vi "RT Simulator.vi"() -> ()   [LabVIEW 2015]
uses:
  Type/RT Loop Events.ctl
  Type/TCP Packet Info.ctl
  Type/_RT Command.ctl
panel:
  out "ms Between Commands":u32
  in  "Stop Button":bool
  out "Read Error":errorcluster
  out "Status":string="PC Communication Established"
  out "Time (s)":dbl
  out "Fault":bool
  out "Ready":bool
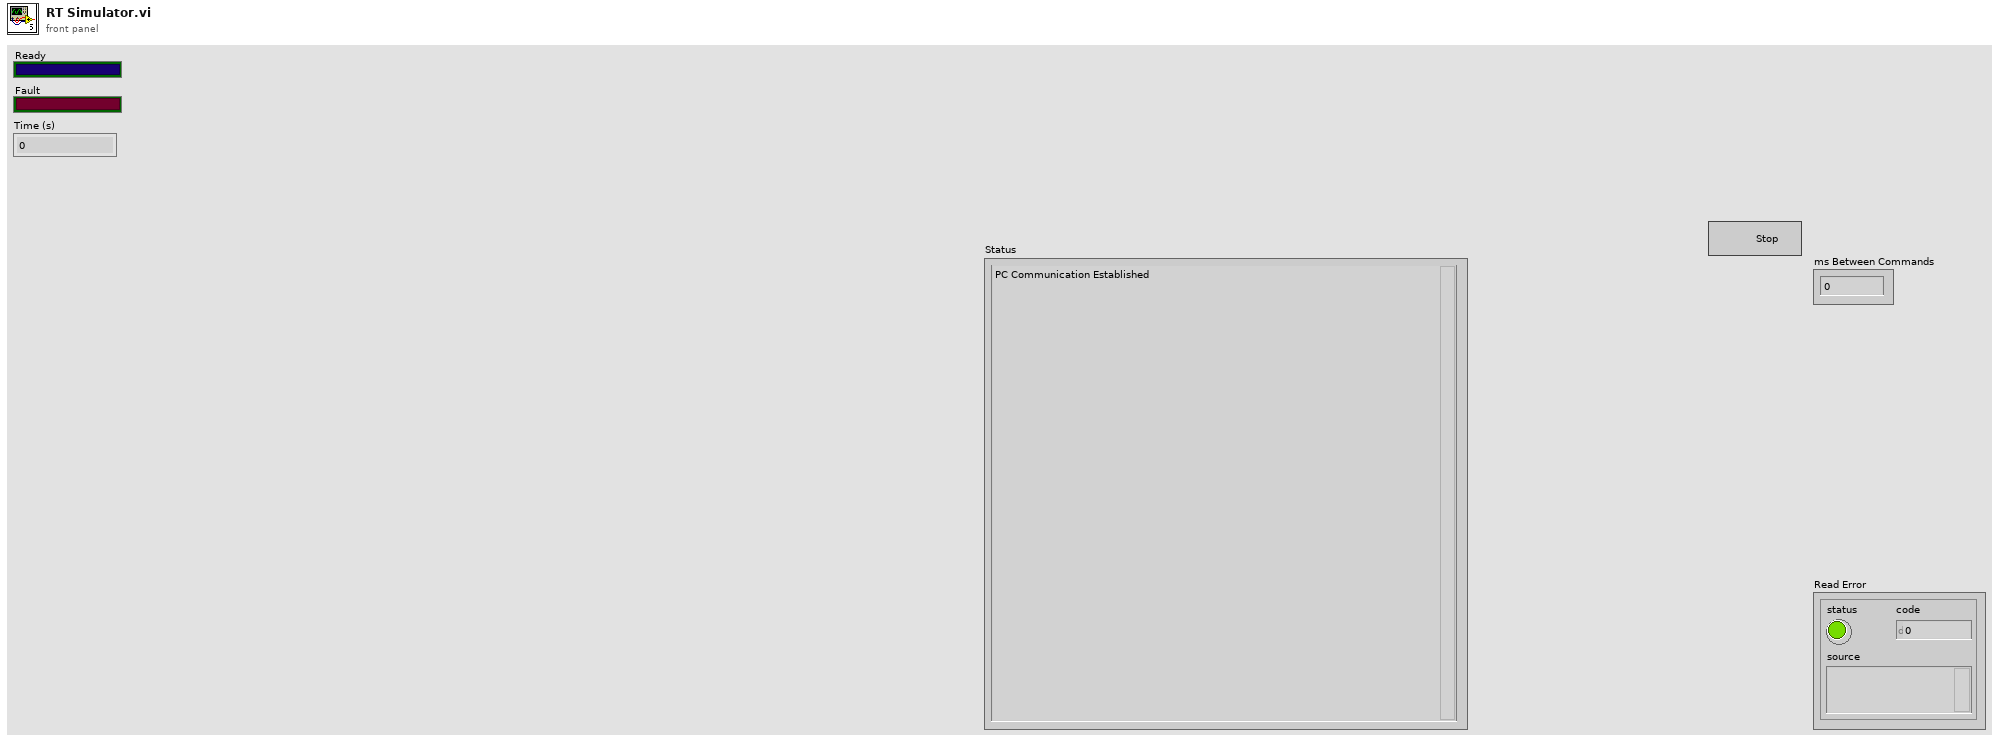
[diagram p1: front panel]
types:
  T1 = typedef "TCP Packet Info.ctl" = cluster{"Packet Signature":string, "Sequence Number":i32, "Command":T2, "Data Message Size":u32, "Data Message Size":string, "Data Message":string, "Error Message Size":u32, "Error Message Size":string, "Error Message":string, "Checksum":u32, "Error Message":errorcluster, "Command ID":string}
  T2 = typedef "_RT Command.ctl" = enum16{"xml Start Run", "xml Start Actual Run", "xml Stop Run", "xml Runtime Update", "xml Get Status", "xml Get Table", "xml Set Table", "xml Get Configuration", "xml System Status", "xml Set LC Input Logic", "xml Get Data", "xml Get Info", "Start", "StartActualRun", "Stop", "Runtime Update", "Get Data", "Get Info", "Get Status", "Get Param", "Get Config", "Get Table", "Read ADC", "Set Oscillator", "Update Config", "Update Table", "Set All Pol", "Set Pol and DC", "Set Max Mass", "Toggle RP", "Toggle EL", "Set PIC", "Initialize Turbo", "Send Turbo Comm", "Close Turbo", "P1", "P2", "P3", "Send Serial", "Set LC Out", "Get LC In", "Read VAC", "Test Table", "Toggle Power", "Get Startup", "Set Startup", "Get ADC Table", "Set ADC Table", "Get Brief Status", "Get Detail Status", "Auxiliary Update", "Set CC Logics", "Set CC Input Logics", "Ignore Error", "invalid"}
  T3 = typedef "RT Loop Events.ctl" = enum16{"Initialize", "Wait for Connection", "Wait for Command", "Send Reply"}
  T4 = cluster{"Rt Loop Events":T3, "Connection ID":refnum<k5>, "error":errorcluster, "Packet Info":T1, "Event":string}
  T5 = enum16{"big-endian, network order", "native, host order", "little-endian"}
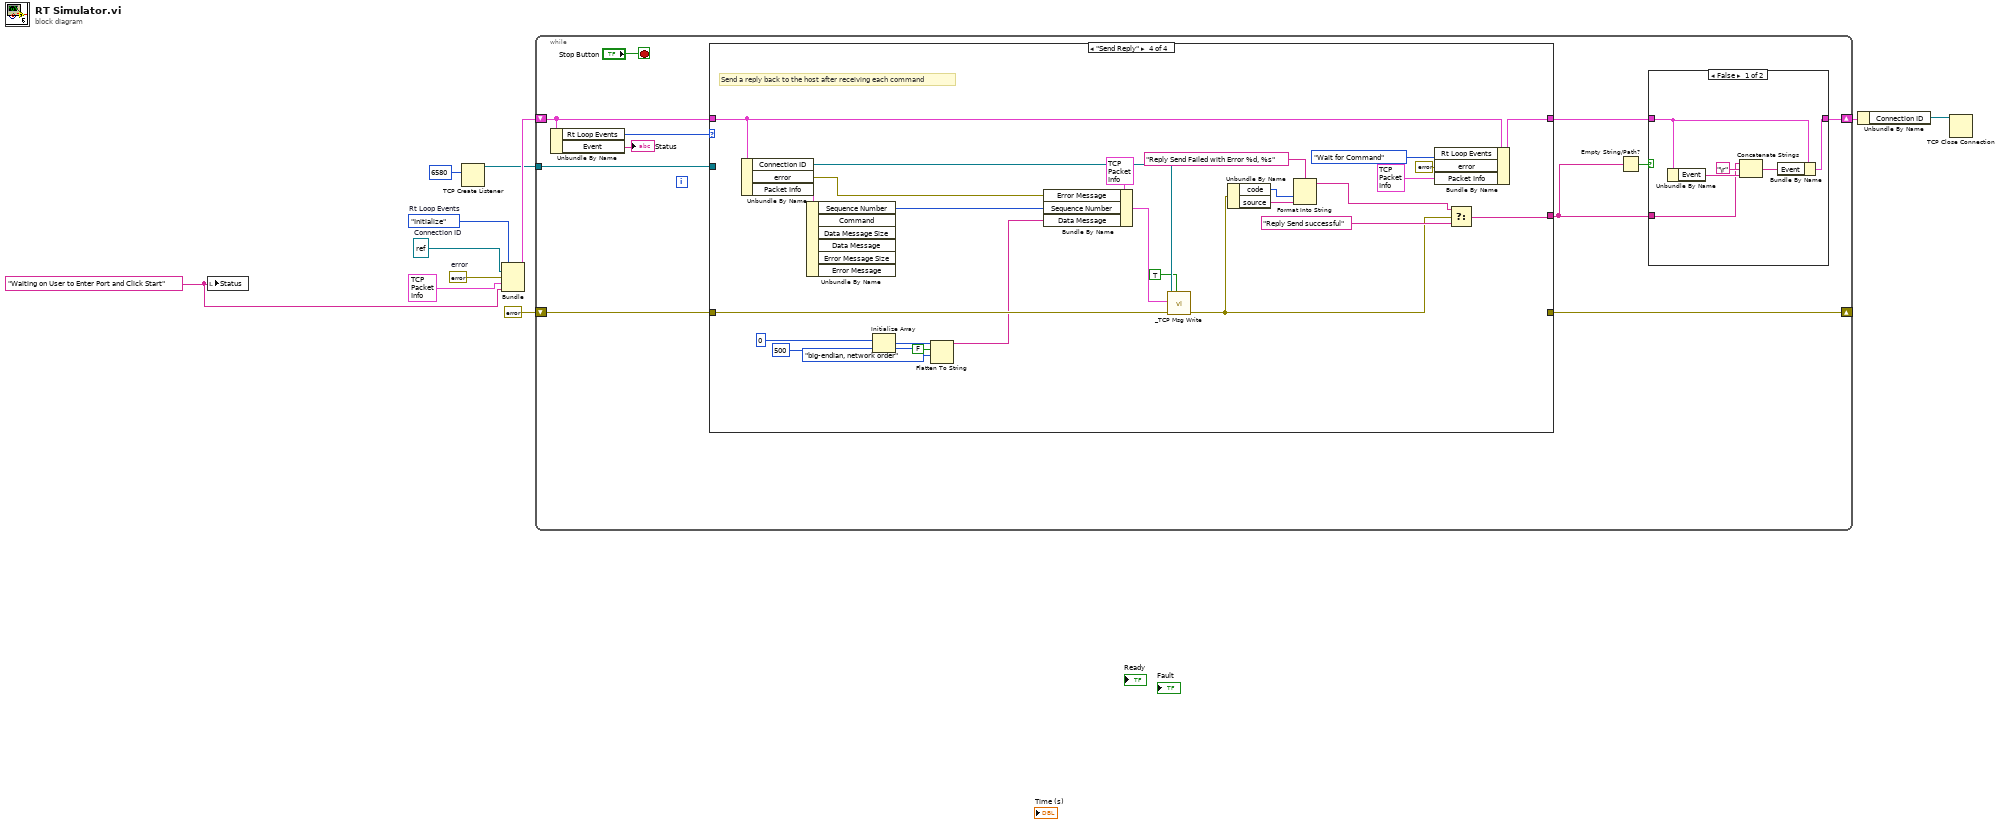
[diagram p0: block diagram]
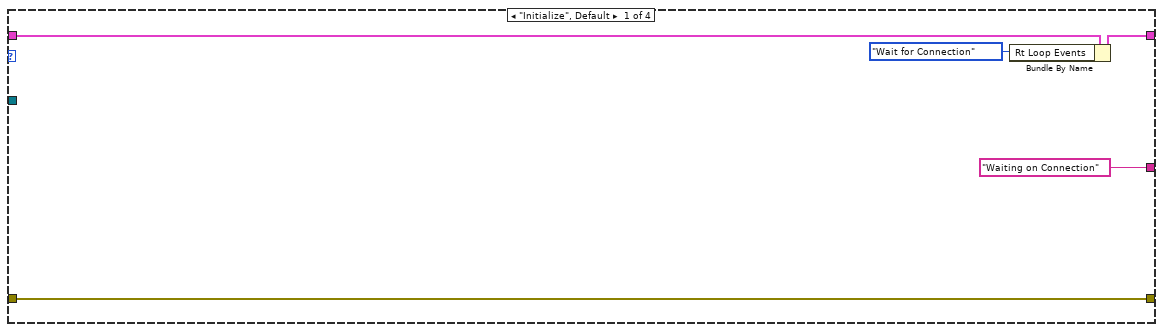
[diagram p3: hidden frame]
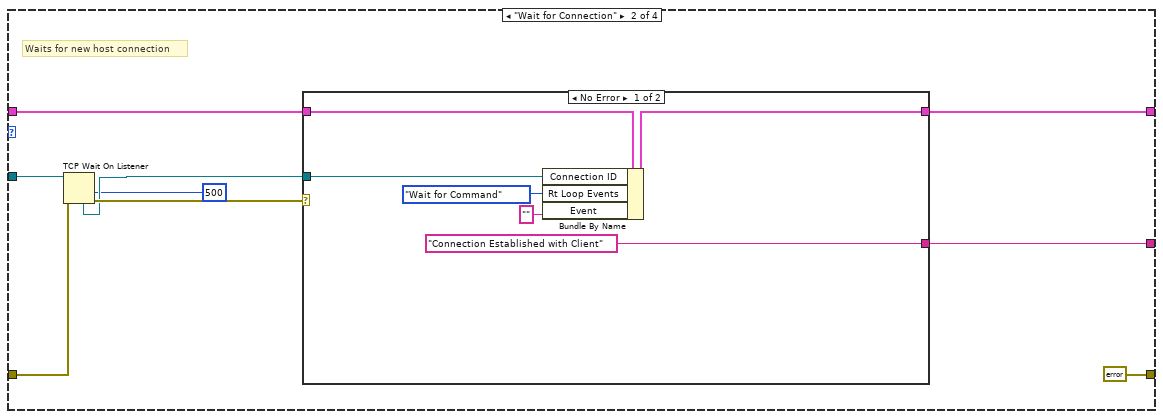
[diagram p4: hidden frame]
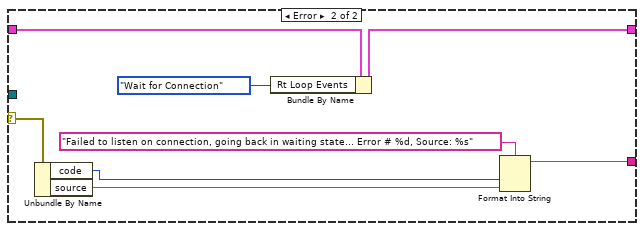
[diagram p5: hidden frame]
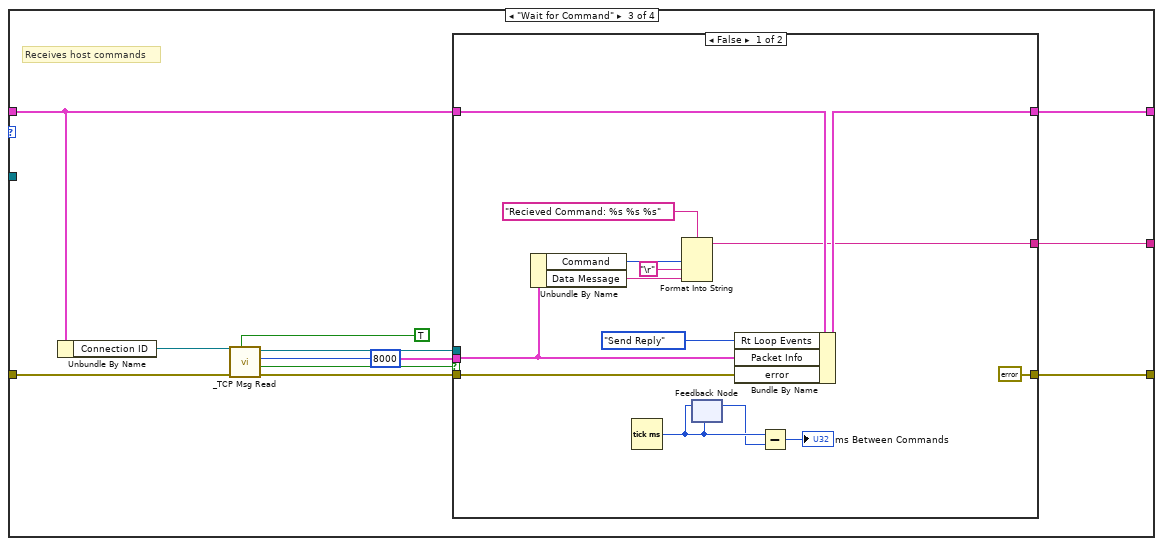
[diagram p6: hidden frame]
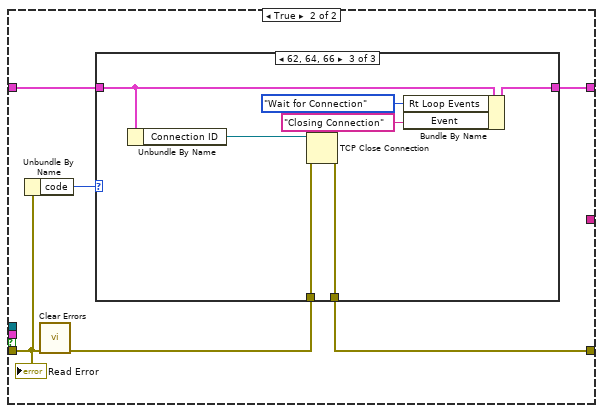
[diagram p7: hidden frame]
diagram:
  w3 = "Waiting on User to Enter Port and Click Start" ("Event")
  w8 = errorcluster {"status"=FALSE, "code"=0, "source"=""}  # error
  w10 = refnum<k5> refnum  # Connection ID
  w11 = RT_Loop_Events."Initialize"  # Rt Loop Events
  n1 = local write "Status"(w3) -> ()
  n2 = TCP Create Listener(10:u16 6580 ("TCP Communication port")) -> (3:w6:refnum<k5>)  [unwired: 1 in, 5 out]
  n3 = Bundle("Rt Loop Events"=w11, "Connection ID"=w10, "error"=w8, "Packet Info"=T1 {"Packet Signature"="", "Sequence Number"=0, "Command"=enum."Get Info", "Data Message Size"=0, "Data Message Size"="", "Data Message"="", "Error Message Size"=0, "Error Message Size"="", "Error Message"="", "Checksum"=0, "Error Message"={"status"=FALSE, "code"=0, "source"=""}, "Command ID"=""}, "Event"=w3) -> (w9:T4)  [unwired: 1 out]
  n4 = while {
    shift-right: [w12] -> w2
    shift-left: w9 -> [w21]
    tunnel: w6 -> [w20]
    shift-right: [w18] -> _
    shift-left: errorcluster {"status"=FALSE, "code"=0, "source"=""} ("error in") -> [w19]
    stop <- "Stop Button" stop-if-true
    n5 = Unbundle By Name(w21) -> ("Rt Loop Events"=w22:T3, "Event"=→"Status":string)
    n6 = case shown="\"Send Reply\"" w22 {
      tunnel: w21 -> [w33 w43 w60 w124]
      tunnel: [w32 w42 w59 w123] -> w13
      tunnel: w20 -> [_ w40 _ _]
      tunnel: w19 -> [w31 w37 w67 w122]
      tunnel: [w31 errorcluster {"status"=FALSE, "code"=0, "source"=""} ("error in") w61 _] -> w18
      tunnel: ["Waiting on Connection" ("Status") w35 w58 w114] -> w15
      frame "Initialize", Default {
        n7 = Bundle By Name(cluster=w33, "Rt Loop Events"=RT_Loop_Events."Wait for Connection") -> (w32:T4)
      }
      frame "Wait for Connection" {
        # "Waits for new host connection"
        n8 = TCP Wait On Listener(8:w37, 9:500 ("timeout ms (wait forever: -1)"), 11:w40) -> (0:w41:errorcluster, 4:w39:refnum<k5>)  [unwired: 4 out]
        n9 = case shown="No Error" w41 {
          selector: w41 -> [_ w54]
          tunnel: w43 -> [w49 w57]
          tunnel: w39 -> [w46 _]
          tunnel: [w48 w55] -> w42
          tunnel: ["Connection Established with Client" ("Event") w52] -> w35
          frame No Error {
            n10 = Bundle By Name(cluster=w49, "Connection ID"=w46, "Rt Loop Events"=RT_Loop_Events."Wait for Command", "Event"="") -> (w48:T4)
          }
          frame Error {
            n11 = Unbundle By Name(w54) -> ("code"=w51:i32, "source"=w50:string)
            n12 = Bundle By Name(cluster=w57, "Rt Loop Events"=RT_Loop_Events."Wait for Connection") -> (w55:T4)
            n13 = Format Into String(format string="Failed to listen on connection, going back in waiting state... Error # %d, Source: %s" ("string"), w51, w50) -> (resulting string=w52:string)  [unwired: 2 in, 1 out]
          }
        }
      }
      frame "Wait for Command" {
        # "Receives host commands"
        n14 = Unbundle By Name(w60) -> ("Connection ID"=w68:refnum<k5>)
        n15 = call "_TCP Msg Read.vi"("RT"=TRUE, "error in"=w67, "timeout ms (10000)"=8000 ("millisecond multiple"), "connection ID"=w68) -> ("error out"=w65:errorcluster, "Read Timeout"=w64:bool, "Packet Info"=w63:T1, "connection ID out"=w62:refnum<k5>)  [unwired: 4 out]
        n16 = case shown="False" w64 {
          tunnel: w65 -> [w80 w89]
          tunnel: w63 -> [w78 _]
          tunnel: w62 -> [_ _]
          tunnel: [errorcluster {"status"=FALSE, "code"=0, "source"=""} ("error out") w84] -> w61
          tunnel: w60 -> [w83 w87]
          tunnel: [w82 w86] -> w59
          tunnel: [w73 _] -> w58
          frame False {
            n17 = Unbundle By Name(w78) -> ("Command"=w77:T2, "Data Message"=w74:string)
            n18 = Tick Count (ms)() -> (millisecond timer value=w72:u32)
            n19 = Format Into String(format string="Recieved Command: %s %s %s", w77, "\r", w74) -> (resulting string=w73:string)  [unwired: 2 in, 1 out]
            n20 = feedback-in #1(w72) -> ()
            n21 = feedback #1(w72) -> (w71:u32)
            n22 = Bundle By Name(cluster=w83, "Rt Loop Events"=RT_Loop_Events."Send Reply", "Packet Info"=w78, "error"=w80) -> (w82:T4)
            n23 = Subtract(x=w72, y=w71) -> (x-y=→"ms Between Commands":u32)
          }
          frame True {
            n24 = Unbundle By Name(w89) -> ("code"=w88:i32)
            n25 = call <vilib>:"Clear Errors.vi"("error in (no error)"=w89) -> ("error out"=w85:errorcluster)  [unwired: 5 in, 1 out]
            n26 = case shown="62, 64, 66" w88 {
              tunnel: w87 -> [w91 w93 w98]
              tunnel: [w91 w93 w100] -> w86
              tunnel: w85 -> [w90 w92 w96]
              tunnel: [w90 w92 w95] -> w84
              frame Default {
              }
              frame 9000.. {
              }
              frame 62, 64, 66 {
                n27 = Unbundle By Name(w98) -> ("Connection ID"=w97:refnum<k5>)
                n28 = TCP Close Connection(connection ID=w97, error in (no error)=w96) -> (error out=w95:errorcluster)  [unwired: 1 in, 1 out]
                n29 = Bundle By Name(cluster=w98, "Rt Loop Events"=RT_Loop_Events."Wait for Connection", "Event"="Closing Connection") -> (w100:T4)
              }
            }
            "Read Error" <- w89
          }
        }
      }
      frame "Send Reply" {
        # "Send a reply back to the host after receiving each command"
        n30 = Unbundle By Name(w124) -> ("Connection ID"=w126:refnum<k5>, "error"=w120:errorcluster, "Packet Info"=w119:T1)
        n31 = Unbundle By Name(w119) -> ("Sequence Number"=w102:i32)  [unwired: 5 out]
        n32 = Initialize Array(0, 500 ("dimension size")) -> (w105:i32[])
        n33 = Flatten To String(anything=w105, prepend array or string size? (T)=FALSE, byte order (0:big-endian, network order)=T5."big-endian, network order") -> (data string=w101:string)  [unwired: 1 in, 2 out]
        n34 = Bundle By Name(cluster=T1 {"Packet Signature"="", "Sequence Number"=0, "Command"=enum."xml Set LC Input Logic", "Data Message Size"=0, "Data Message Size"="", "Data Message"="", "Error Message Size"=0, "Error Message Size"="", "Error Message"="", "Checksum"=0, "Error Message"={"status"=FALSE, "code"=0, "source"=""}, "Command ID"=""} ("Packet Info In"), "Error Message"=w120, "Sequence Number"=w102, "Data Message"=w101) -> (w118:T1)
        n35 = call "_TCP Msg Write.vi"("RT"=TRUE, "error in"=w122, "Packet Info In"=w118, "connection ID In"=w126) -> ("error out 2"=w111:errorcluster)  [unwired: 1 in, 6 out]
        n36 = Unbundle By Name(w111) -> ("code"=w113:i32, "source"=w112:string)
        n37 = Format Into String(format string="Reply Send Failed with Error %d, %s", w113, w112) -> (resulting string=w109:string)  [unwired: 2 in, 1 out]
        n38 = Bundle By Name(cluster=w124, "Rt Loop Events"=RT_Loop_Events."Wait for Command", "error"=errorcluster {"status"=FALSE, "code"=0, "source"=""}, "Packet Info"=T1 {"Packet Signature"="", "Sequence Number"=0, "Command"=enum."Get Info", "Data Message Size"=0, "Data Message Size"="", "Data Message"="", "Error Message Size"=0, "Error Message Size"="", "Error Message"="", "Checksum"=0, "Error Message"={"status"=FALSE, "code"=0, "source"=""}, "Command ID"=""}) -> (w123:T4)
        n39 = Select(t=w109, s=w111, f="Reply Send successful" ("Event")) -> (s? t:f=w114:string)
      }
    }
    n40 = Empty String/Path?(string/path=w15) -> (empty?=w14:bool)
    n41 = case shown="False" w14 {
      tunnel: w15 -> [w23 _]
      tunnel: w13 -> [w27 w29]
      tunnel: [w26 w29] -> w12
      frame False {
        n42 = Unbundle By Name(w27) -> ("Event"=w24:string)
        n43 = Concatenate Strings(w23, "\r", w24) -> (w28:string)
        n44 = Bundle By Name(cluster=w27, "Event"=w28) -> (w26:T4)
      }
      frame True {
      }
    }
  }
  n45 = Unbundle By Name(w2) -> ("Connection ID"=w1:refnum<k5>)
  n46 = TCP Close Connection(connection ID=w1) -> ()  [unwired: 2 in, 2 out]
